vi "Pi_I2C_BMP280_Temp.vi"() -> ()   [LabVIEW 2020, in "BMP208.lvclass"]
uses:
  BMP208.lvclass
  Controls/td_enum_powermode.ctl
  Controls/td_enum_osrsX.ctl
  Controls/td_cluster_Temp_Coeff.ctl
  <vilib>/MakerHub/LINX/Private/Local IO/LinxI2cWrite.vi
  <vilib>/MakerHub/LINX/Public/Utilities/Check Channel.vi
  <vilib>/MakerHub/LINX/Private/Local IO/Handle Errors.vi
  <vilib>/MakerHub/LINX/Public/Utilities/Open Local.vi
  <vilib>/MakerHub/LINX/Private/Utilties/Generate Error.vi
  <vilib>/MakerHub/LINX/LMH-LINX.lvlib
panel:
  out "T3":u16
  out "T2":u16
  out "T1":u16
  out "Temp":dbl
  out "Temperature 2":u32 format="%020b"
  in  "stop":bool
  out "ctrl_meas":u8[](array[numeric]) format="%08b"
  out "Temperature":u8[](array[numeric]) format="%08b"
  out "Pressure":u8[](array[numeric]) format="%08b"
  out "Status":u8[](array[numeric]) format="%08b"
  out "Device Name":string
  out "ChipID":u8[](array[numeric]) format="%02x"
  out "error out":errorcluster
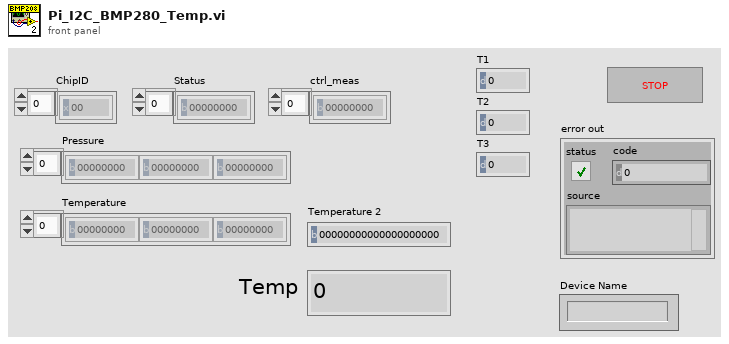
[diagram p1: front panel]
types:
  T1 = typedef "BMP208.lvclass/td_cluster_Temp_Coeff.ctl" = cluster{"T1":u16, "T2":i16, "T3":i16}
  T2 = typedef "BMP208.lvclass/td_enum_osrsX.ctl" = enum16{"Skipped", "16b", "17b", "18b", "19b", "20b", "20b_2", "20b_3"}
  T3 = typedef "BMP208.lvclass/td_enum_powermode.ctl" = enum16{"Sleep", "Forced", "Forced_", "Normal"}
  T4 = typedef "LMH-LINX.lvlib/LINX Ref.ctl" = cluster{"IO":T5, "Interface":T6, "LINX Device Config":T7}
  T5 = typedef "LMH-LINX.lvlib/Platform.ctl" = enum16{"Remote", "Local"}
  T6 = typedef "LMH-LINX.lvlib/Interface.ctl" = enum16{"Serial", "TCP"}
  T7 = typedef "LMH-LINX.lvlib/Device.lvlib/LINX Device Config.ctl" = cluster{"Interface":T6, "COM Port":refnum<visa-resource-name>, "TCP Configuration":T8, "Device Family":u8, "Device ID":u8, "Device Name":string, "TCP Ref":refnum<k5>, "Channels":T9}
  T8 = typedef "LMH-LINX.lvlib/Device.lvlib/TCP Config.ctl" = cluster{"IP Address":string, "Port":u16}
  T9 = typedef "LMH-LINX.lvlib/Channels.ctl" = cluster{"DI":u8[], "DO":u8[], "AI":u8[], "AO":u8[], "PWM":u8[], "QE":u8[], "UART":u8[], "I2C 2":u8[], "SPI":u8[], "CAN":u8[], "Servo":u8[], "AI Ref (V)":dbl, "AI Resolution (Bits)":u8, "AO Ref (V)":dbl, "AO Resolution (Bits)":u8}
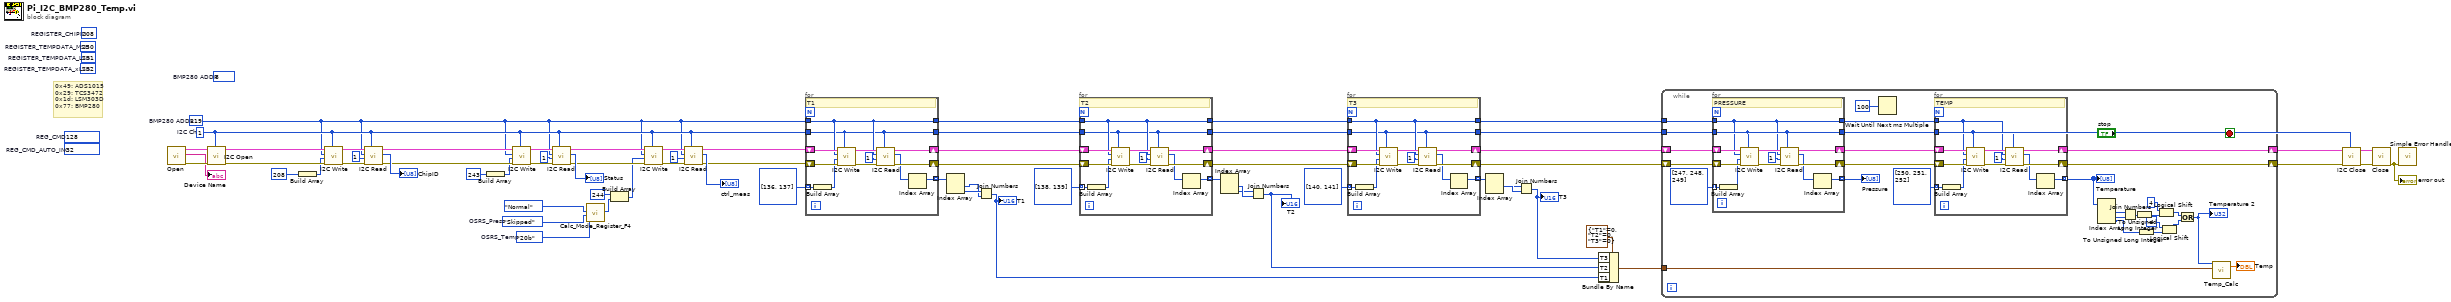
[diagram p0: block diagram]
diagram:
  w7 = td_enum_osrsX."Skipped"  # OSRS_Press
  w6 = td_enum_osrsX."20b"  # OSRS_Temp
  (unwired) u8 8  # BMP280 ADDR
  (unwired) u8 208  # REGISTER_CHIPID
  (unwired) u8 252  # REGISTER_TEMPDATA_xLSB
  (unwired) u8 251  # REGISTER_TEMPDATA_LSB
  (unwired) u8 250  # REGISTER_TEMPDATA_MSB
  w36 = u8 119  # BMP280 ADDR
  w37 = u8 1  # I2C Ch
  (unwired) u8 128  # REG_CMD
  (unwired) u8 32  # REG_CMD_AUTO_INC
  # "0x49: ADS1015\n0x29: TCS3472\n0x1d: LSM303D\n0x77: BMP280"
  n1 = call-poly <vilib>:"Open.vi"() -> ("Error Out"=w69:errorcluster, "Device Name"=→"Device Name":string, "LINX Resource"=w67:T4)  [unwired: 9 in]
  n2 = call <vilib>:"I2C Open.vi"("I2C Channel (0)"=w37, "Error In"=w69, "LINX Resource"=w67) -> ("Error Out"=w68:errorcluster, "LINX Resource"=w59:T4)  [unwired: 7 in]
  n3 = Build Array(u8 208 ("I2C Slave Address 2")) -> (w56:u8[])
  n4 = call <vilib>:"I2C Write.vi"("I2C Channel"=w37, "Error In"=w68, "Data"=w56, "I2C Slave Address (0)"=w36, "LINX Resource"=w59) -> ("Error Out"=w60:errorcluster, "LINX Resource"=w58:T4)  [unwired: 5 in]
  n5 = call <vilib>:"I2C Read.vi"("I2C Channel"=w37, "Error In"=w60, "Bytes To Read"=u8 1, "I2C Slave Address (0)"=w36, "LINX Resource"=w58) -> ("Error Out"=w53:errorcluster, "Data"=→"ChipID":u8[], "LINX Resource"=w54:T4)  [unwired: 4 in]
  n6 = Build Array(u8 243 ("I2C Slave Address 2")) -> (w49:u8[])
  n7 = call <vilib>:"I2C Write.vi"("I2C Channel"=w37, "Error In"=w53, "Data"=w49, "I2C Slave Address (0)"=w36, "LINX Resource"=w54) -> ("Error Out"=w51:errorcluster, "LINX Resource"=w52:T4)  [unwired: 5 in]
  n8 = call <vilib>:"I2C Read.vi"("I2C Channel"=w37, "Error In"=w51, "Bytes To Read"=u8 1, "I2C Slave Address (0)"=w36, "LINX Resource"=w52) -> ("Error Out"=w43:errorcluster, "Data"=→"Status":u8[], "LINX Resource"=w44:T4)  [unwired: 4 in]
  n9 = call "Calc_Mode_Register_F4.vi"("OSRS_Temp"=w6, "OSRS_Press"=w7, "PowerMode"=td_enum_powermode."Normal") -> ("F4_Register"=w9:u8)  [unwired: 8 in]
  n10 = Build Array(u8 244 ("I2C Slave Address 2"), w9) -> (w40:u8[])
  n11 = call <vilib>:"I2C Write.vi"("I2C Channel"=w37, "Error In"=w43, "Data"=w40, "I2C Slave Address (0)"=w36, "LINX Resource"=w44) -> ("Error Out"=w45:errorcluster, "LINX Resource"=w42:T4)  [unwired: 5 in]
  n12 = call <vilib>:"I2C Read.vi"("I2C Channel"=w37, "Error In"=w45, "Bytes To Read"=u8 1, "I2C Slave Address (0)"=w36, "LINX Resource"=w42) -> ("Error Out"=w15:errorcluster, "Data"=→"ctrl_meas":u8[], "LINX Resource"=w17:T4)  [unwired: 4 in]
  n13 = for {
    tunnel: [w72] -> w26 mode=indexing
    tunnel: u8[] [136, 137] ("Data") -> [w75] mode=indexing
    tunnel: w37 -> [w70]
    tunnel: w36 -> [w71]
    shift-right: [w77] -> w16
    shift-left: w17 -> [w80]
    shift-right: [w76] -> w14
    shift-left: w15 -> [w79]
    tunnel: [w71] -> w35
    tunnel: [w70] -> w32
    # "T1"
    n14 = Build Array(w75) -> (w74:u8[])
    n15 = call <vilib>:"I2C Write.vi"("I2C Channel"=w70, "Error In"=w79, "Data"=w74, "I2C Slave Address (0)"=w71, "LINX Resource"=w80) -> ("Error Out"=w82:errorcluster, "LINX Resource"=w78:T4)  [unwired: 5 in]
    n16 = call <vilib>:"I2C Read.vi"("I2C Channel"=w70, "Error In"=w82, "Bytes To Read"=u8 1, "I2C Slave Address (0)"=w71, "LINX Resource"=w78) -> ("Error Out"=w76:errorcluster, "Data"=w73:u8[], "LINX Resource"=w77:T4)  [unwired: 4 in]
    n17 = Index Array(array=w73) -> (element=w72:u8)  [unwired: 1 in]
  }
  n18 = Index Array(array=w26) -> (element #1=w22:u8, element #2=w23:u8)  [unwired: 2 in]
  n19 = Join Numbers(hi=w23, lo=w22) -> ((hi.lo)=w2:u16)
  "T1" <- w2
  n20 = for {
    tunnel: [w85] -> w25 mode=indexing
    tunnel: u8[] [138, 139] ("Data") -> [w88] mode=indexing
    tunnel: w32 -> [w83]
    tunnel: w35 -> [w84]
    shift-right: [w90] -> w12
    shift-left: w16 -> [w93]
    shift-right: [w89] -> w13
    shift-left: w14 -> [w92]
    tunnel: [w84] -> w34
    tunnel: [w83] -> w31
    # "T2"
    n21 = Build Array(w88) -> (w87:u8[])
    n22 = call <vilib>:"I2C Write.vi"("I2C Channel"=w83, "Error In"=w92, "Data"=w87, "I2C Slave Address (0)"=w84, "LINX Resource"=w93) -> ("Error Out"=w95:errorcluster, "LINX Resource"=w91:T4)  [unwired: 5 in]
    n23 = call <vilib>:"I2C Read.vi"("I2C Channel"=w83, "Error In"=w95, "Bytes To Read"=u8 1, "I2C Slave Address (0)"=w84, "LINX Resource"=w91) -> ("Error Out"=w89:errorcluster, "Data"=w86:u8[], "LINX Resource"=w90:T4)  [unwired: 4 in]
    n24 = Index Array(array=w86) -> (element=w85:u8)  [unwired: 1 in]
  }
  n25 = Index Array(array=w25) -> (element #1=w21:u8, element #2=w20:u8)  [unwired: 2 in]
  n26 = Join Numbers(hi=w20, lo=w21) -> ((hi.lo)=w3:u16)
  "T2" <- w3
  n27 = for {
    tunnel: [w98] -> w24 mode=indexing
    tunnel: u8[] [140, 141] ("Data") -> [w101] mode=indexing
    tunnel: w31 -> [w96]
    tunnel: w34 -> [w97]
    shift-right: [w103] -> w11
    shift-left: w12 -> [w106]
    shift-right: [w102] -> w10
    shift-left: w13 -> [w105]
    tunnel: [w97] -> w33
    tunnel: [w96] -> w30
    # "T3"
    n28 = Build Array(w101) -> (w100:u8[])
    n29 = call <vilib>:"I2C Write.vi"("I2C Channel"=w96, "Error In"=w105, "Data"=w100, "I2C Slave Address (0)"=w97, "LINX Resource"=w106) -> ("Error Out"=w108:errorcluster, "LINX Resource"=w104:T4)  [unwired: 5 in]
    n30 = call <vilib>:"I2C Read.vi"("I2C Channel"=w96, "Error In"=w108, "Bytes To Read"=u8 1, "I2C Slave Address (0)"=w97, "LINX Resource"=w104) -> ("Error Out"=w102:errorcluster, "Data"=w99:u8[], "LINX Resource"=w103:T4)  [unwired: 4 in]
    n31 = Index Array(array=w99) -> (element=w98:u8)  [unwired: 1 in]
  }
  n32 = Index Array(array=w24) -> (element #1=w19:u8, element #2=w18:u8)  [unwired: 2 in]
  n33 = Join Numbers(hi=w18, lo=w19) -> ((hi.lo)=w4:u16)
  "T3" <- w4
  n34 = Bundle By Name(cluster=T1 {"T1"=0, "T2"=0, "T3"=0} ("TempCoeff"), "T3"=w4, "T2"=w3, "T1"=w2) -> (w1:T1)
  n35 = while {
    tunnel: w30 -> [w129]
    tunnel: w33 -> [w128]
    shift-right: [w135] -> w47
    shift-left: w11 -> [w131]
    shift-right: [w134] -> w46
    shift-left: w10 -> [w130]
    tunnel: w1 -> [w109]
    stop <- "stop" stop-if-true
    n36 = for {
      tunnel: [w153] -> w125 mode=indexing
      tunnel: u8[] [247, 248, 249] ("Data") -> [w158] mode=indexing
      tunnel: w129 -> [w151]
      tunnel: w128 -> [w152]
      shift-right: [w160] -> w137
      shift-left: w131 -> [w157]
      shift-right: [w159] -> w136
      shift-left: w130 -> [w156]
      tunnel: [w152] -> w122
      tunnel: [w151] -> w121
      # "PRESSURE"
      n37 = Build Array(w158) -> (w155:u8[])
      n38 = call <vilib>:"I2C Write.vi"("I2C Channel"=w151, "Error In"=w156, "Data"=w155, "I2C Slave Address (0)"=w152, "LINX Resource"=w157) -> ("Error Out"=w162:errorcluster, "LINX Resource"=w161:T4)  [unwired: 5 in]
      n39 = call <vilib>:"I2C Read.vi"("I2C Channel"=w151, "Error In"=w162, "Bytes To Read"=u8 1, "I2C Slave Address (0)"=w152, "LINX Resource"=w161) -> ("Error Out"=w159:errorcluster, "Data"=w154:u8[], "LINX Resource"=w160:T4)  [unwired: 4 in]
      n40 = Index Array(array=w154) -> (element=w153:u8)  [unwired: 1 in]
    }
    "Pressure" <- w125
    n41 = Wait Until Next ms Multiple(millisecond multiple=u32 100) -> ()  [unwired: 1 out]
    n42 = for {
      tunnel: [w138] -> w124 mode=indexing
      tunnel: u8[] [250, 251, 252] ("Data") -> [w143] mode=indexing
      tunnel: w121 -> [w142]
      tunnel: w122 -> [w141]
      shift-right: [w145] -> w135
      shift-left: w137 -> [w148]
      shift-right: [w144] -> w134
      shift-left: w136 -> [w147]
      # "TEMP"
      n43 = Build Array(w143) -> (w140:u8[])
      n44 = call <vilib>:"I2C Write.vi"("I2C Channel"=w142, "Error In"=w147, "Data"=w140, "I2C Slave Address (0)"=w141, "LINX Resource"=w148) -> ("Error Out"=w150:errorcluster, "LINX Resource"=w146:T4)  [unwired: 5 in]
      n45 = call <vilib>:"I2C Read.vi"("I2C Channel"=w142, "Error In"=w150, "Bytes To Read"=u8 1, "I2C Slave Address (0)"=w141, "LINX Resource"=w146) -> ("Error Out"=w144:errorcluster, "Data"=w139:u8[], "LINX Resource"=w145:T4)  [unwired: 4 in]
      n46 = Index Array(array=w139) -> (element=w138:u8)  [unwired: 1 in]
    }
    "Temperature" <- w124
    n47 = Index Array(array=w124) -> (element #1=w123:u8, element #2=w118:u8, element #3=w113:u8)  [unwired: 3 in]
    n48 = Join Numbers(hi=w123, lo=w118) -> ((hi.lo)=w120:u16)
    n49 = To Unsigned Long Integer(number=w120) -> (unsigned 32bit integer=w115:u32)
    n50 = To Unsigned Long Integer(number=w113) -> (unsigned 32bit integer=w112:u32)
    n51 = Logical Shift(y=i16 4, x=w115) -> (x << y=w117:u32)
    n52 = Logical Shift(y=i16 -4, x=w112) -> (x << y=w111:u32)
    n53 = Or(x=w117, y=w111) -> (x .or. y?=w114:u32)
    "Temperature 2" <- w114
    n54 = call "Temp_Calc.vi"("TempCoeff"=w109, "raw_temp"=w114) -> ("Temperature"=→"Temp":dbl)  [unwired: 8 in, 1 out]
  }
  n55 = call <vilib>:"I2C Close.vi"("I2C Channel (0)"=w30, "Error In"=w46, "LINX Resource"=w47) -> ("Error Out"=w66:errorcluster, "LINX Resource"=w65:T4)  [unwired: 7 in]
  n56 = call <vilib>:"Close.vi"("Error In"=w66, "LINX Resource"=w65) -> ("Error Out"=w64:errorcluster)  [unwired: 9 in]
  "error out" <- w64
  n57 = call <vilib>:"Simple Error Handler.vi"("error in (no error)"=w64) -> ()  [unwired: 4 in, 5 out]
